vi "LabJack_galvo.vi"() -> ()   [LabVIEW 2025]
uses:
  <vilib>/measure/NI_MABase.lvlib
panel:
  in  "offset":dbl=2.5000000000000013 min=0.0 max=4.5 step=0.1
  in  "stop  2":bool
  in  "stop":bool
  out "DAQ Output Voltage":waveform(dbl)[](graph)
  in  "Waveform Y-Axis":string(combo)="sine"
  in  "Frequency (Hz) 2":i32=20
  in  "Phase (degrees) 2":i32
  in  "Voltage Amplitude 2":dbl=1.0 min=0.0 max=4.5 step=0.1
  in  "Number of Points":dbl=1000.0 format="%#_13g"
  in  "Sampling frequency":dbl=5000.0 format="%#_13g"
  in  "Voltage Amplitude":dbl=1.0 min=0.0 max=4.5 step=0.1
  in  "Phase (degrees)":i32
  in  "Frequency (Hz)":i32=20
  in  "Waveform X-Axis":string(combo)="sine"
  in  "Stream Targets":string[](array[string])=["DAC0", "DAC1"]
  in  "Identifier":string="LJM_idANY"
  in  "ConnectionType":string="LJM_ctANY"
  in  "DeviceType":string="LJM_dtANY"
  out "Error Message":string="No Error"
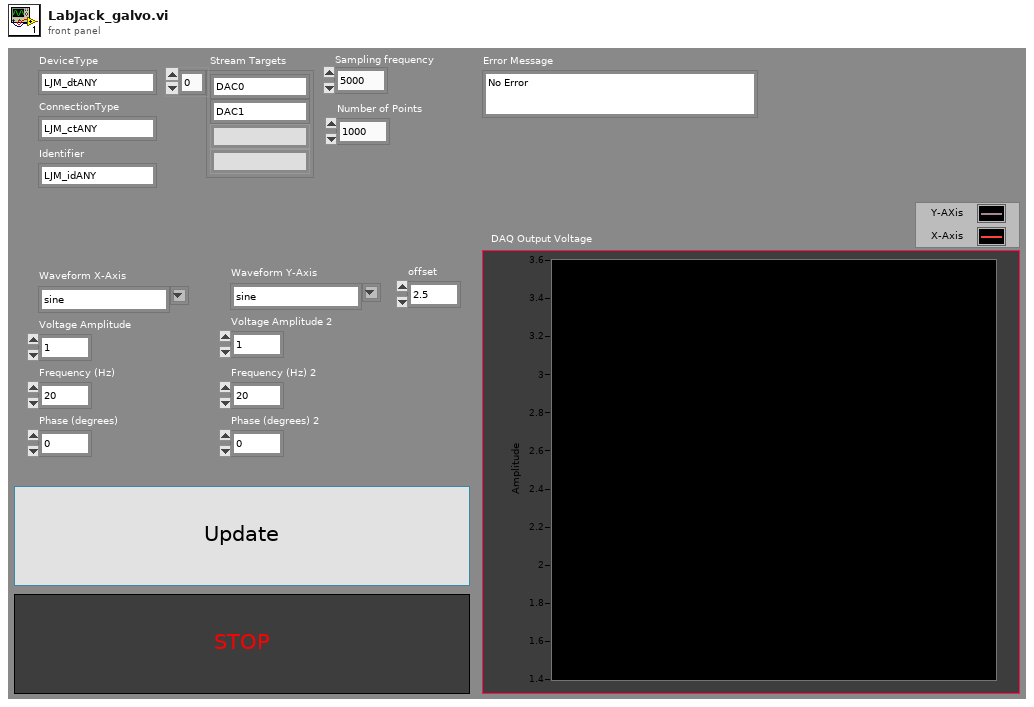
[diagram p1: front panel]
types:
  T1 = cluster{"Sampling frequency":dbl, "Number of Points":dbl}
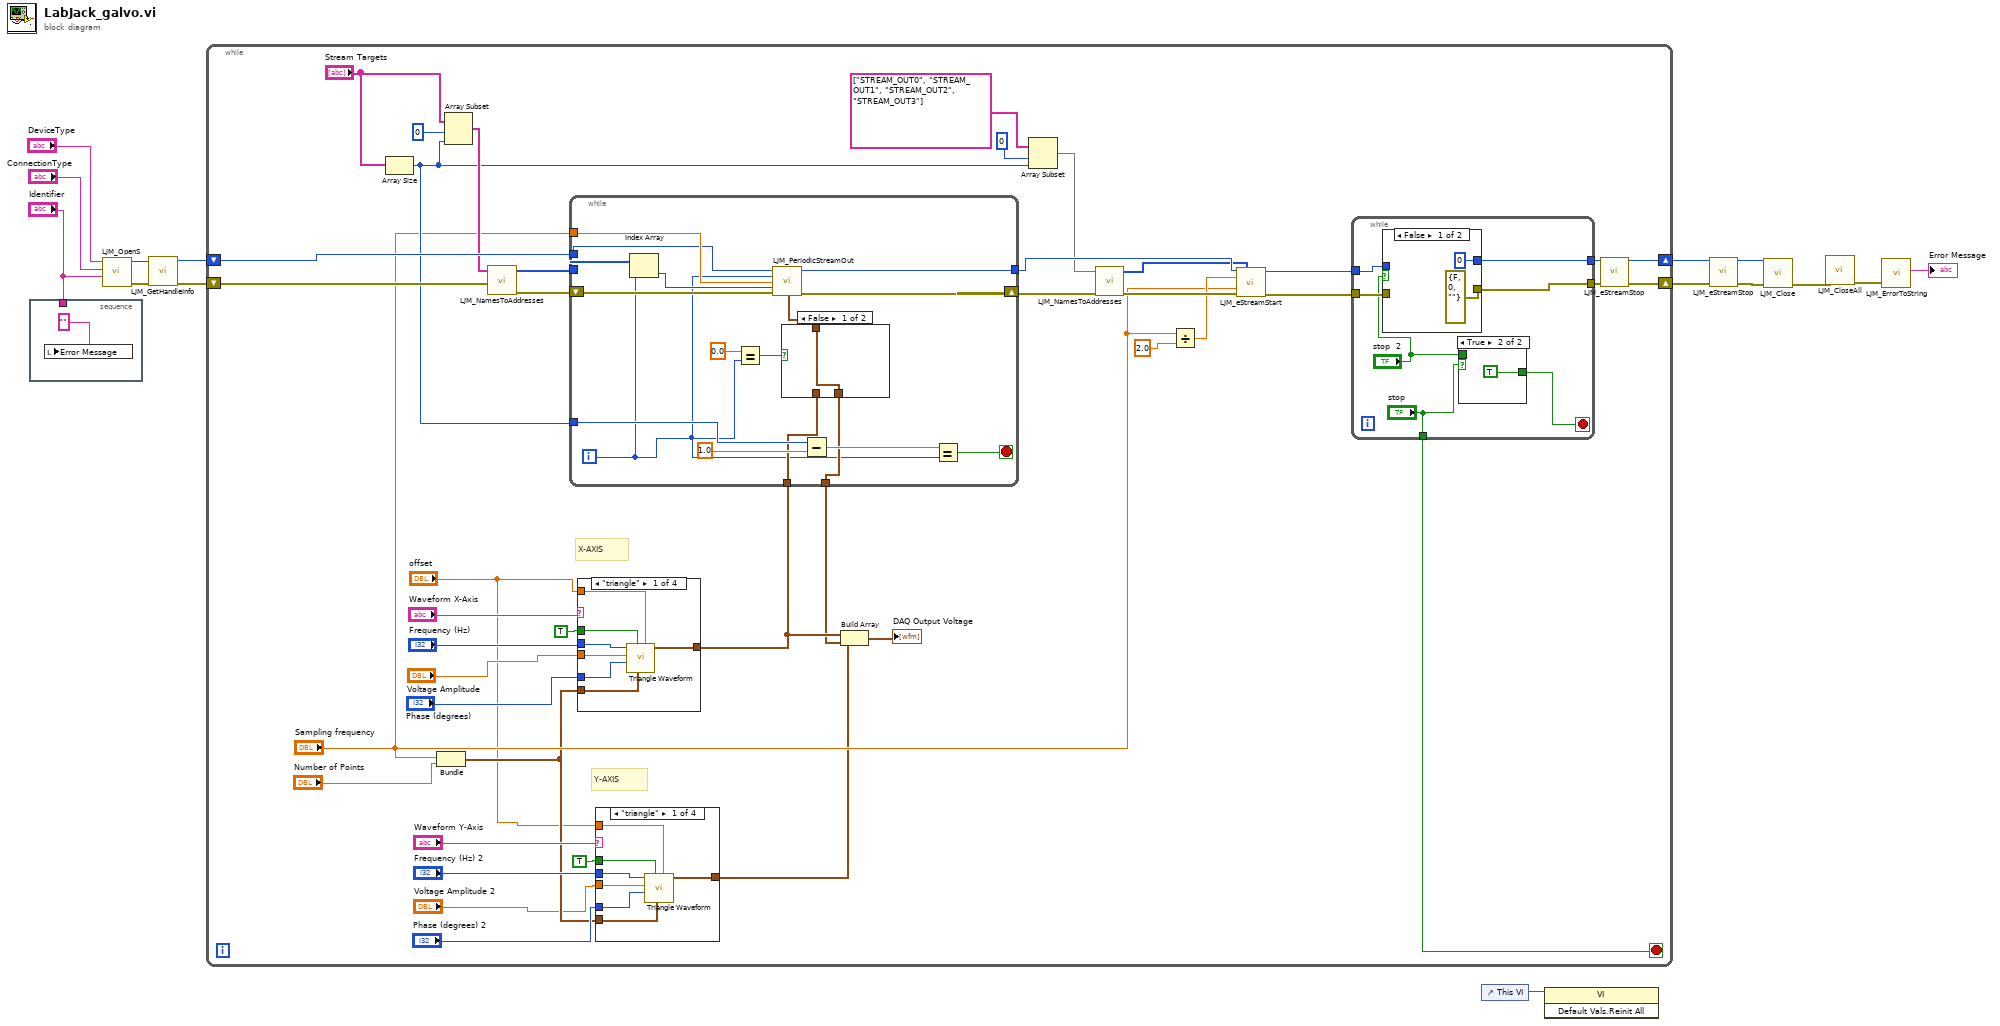
[diagram p0: block diagram]
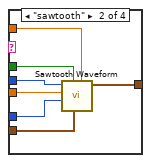
[diagram p4: hidden frame]
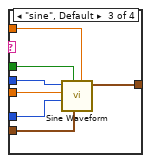
[diagram p5: hidden frame]
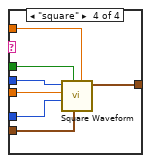
[diagram p6: hidden frame]
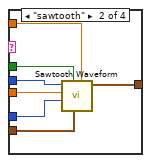
[diagram p7: hidden frame]
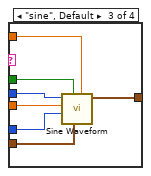
[diagram p8: hidden frame]
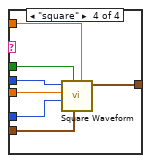
[diagram p9: hidden frame]
diagram:
  n1 = stacked-sequence {
    tunnel: "Identifier" -> [_]
    frame #0 {
      n2 = local write "Error Message"("" ("Error Message")) -> ()
    }
  }
  n3 = call <vilib>:"LJM_OpenS.vi"("Identifier"="Identifier", "ConnectionType"="ConnectionType", "DeviceType"="DeviceType") -> ("error out"=w15:errorcluster, "Handle"=w12:i32)  [unwired: 7 in]
  n4 = call <vilib>:"LJM_GetHandleInfo.vi"("error in"=w15, "Handle In"=w12) -> ("error out"=w9:errorcluster, "Handle Out"=w10:i32)  [unwired: 2 in, 6 out]
  n5 = while {
    shift-right: [w42] -> w4
    shift-left: w10 -> [w56]
    shift-right: [w43] -> w3
    shift-left: w9 -> [w50]
    stop <- w20 stop-if-true
    # "Y-AXIS"
    # "X-AXIS"
    n6 = Array Size(array="Stream Targets") -> (size(s)=w39:i32)
    n7 = Bundle("Sampling frequency"="Sampling frequency", "Number of Points"="Number of Points") -> (w28:T1)  [unwired: 1 in]
    n8 = Array Subset(array="Stream Targets", index=0, length=w39) -> (w53:string[])
    n9 = call <vilib>:"LJM_NamesToAddresses.vi"("error in"=w50, "aNames"=w53) -> ("error out"=w51:errorcluster, "aAddresses"=w52:i32[])  [unwired: 7 in, 1 out]
    n10 = case shown="\"triangle\"" "Waveform X-Axis" {
      tunnel: "Voltage Amplitude" -> [w100 w107 w114 w121]
      tunnel: "Frequency (Hz)" -> [w105 w112 w119 w126]
      tunnel: w28 -> [w102 w109 w117 w125]
      tunnel: [w103 w108 w116 w124] -> w22
      tunnel: "Phase (degrees)" -> [w104 w111 w118 w123]
      tunnel: TRUE ("reset signal") -> [w101 w110 w115 w122]
      tunnel: "offset" -> [w99 w106 w113 w120]
      frame "triangle" {
        n11 = call <vilib>:"Triangle Waveform.vi"("offset"=w99, "sampling info"=w102, "reset signal"=w101, "phase"=w104, "amplitude"=w100, "frequency"=w105) -> ("signal out"=w103:waveform(dbl))  [unwired: 4 in, 1 out]
      }
      frame "sawtooth" {
        n12 = call <vilib>:"Sawtooth Waveform.vi"("offset"=w106, "sampling info"=w109, "reset signal"=w110, "phase"=w111, "amplitude"=w107, "frequency"=w112) -> ("signal out"=w108:waveform(dbl))  [unwired: 4 in, 1 out]
      }
      frame "sine", Default {
        n13 = call <vilib>:"Sine Waveform.vi"("offset"=w113, "sampling info"=w117, "reset signal"=w115, "phase"=w118, "amplitude"=w114, "frequency"=w119) -> ("signal out"=w116:waveform(dbl))  [unwired: 4 in, 1 out]
      }
      frame "square" {
        n14 = call <vilib>:"Square Waveform.vi"("offset"=w120, "sampling info"=w125, "reset signal"=w122, "phase"=w123, "amplitude"=w121, "frequency"=w126) -> ("signal out"=w124:waveform(dbl))  [unwired: 4 in, 1 out]
      }
    }
    n15 = case shown="\"triangle\"" "Waveform Y-Axis" {
      tunnel: "Voltage Amplitude 2" -> [w72 w79 w86 w93]
      tunnel: "Frequency (Hz) 2" -> [w77 w84 w91 w98]
      tunnel: w28 -> [w74 w81 w89 w97]
      tunnel: [w75 w80 w88 w96] -> w21
      tunnel: "Phase (degrees) 2" -> [w76 w83 w90 w95]
      tunnel: TRUE ("reset signal") -> [w73 w82 w87 w94]
      tunnel: "offset" -> [w71 w78 w85 w92]
      frame "triangle" {
        n16 = call <vilib>:"Triangle Waveform.vi"("offset"=w71, "sampling info"=w74, "reset signal"=w73, "phase"=w76, "amplitude"=w72, "frequency"=w77) -> ("signal out"=w75:waveform(dbl))  [unwired: 4 in, 1 out]
      }
      frame "sawtooth" {
        n17 = call <vilib>:"Sawtooth Waveform.vi"("offset"=w78, "sampling info"=w81, "reset signal"=w82, "phase"=w83, "amplitude"=w79, "frequency"=w84) -> ("signal out"=w80:waveform(dbl))  [unwired: 4 in, 1 out]
      }
      frame "sine", Default {
        n18 = call <vilib>:"Sine Waveform.vi"("offset"=w85, "sampling info"=w89, "reset signal"=w87, "phase"=w90, "amplitude"=w86, "frequency"=w91) -> ("signal out"=w88:waveform(dbl))  [unwired: 4 in, 1 out]
      }
      frame "square" {
        n19 = call <vilib>:"Square Waveform.vi"("offset"=w92, "sampling info"=w97, "reset signal"=w94, "phase"=w95, "amplitude"=w93, "frequency"=w98) -> ("signal out"=w96:waveform(dbl))  [unwired: 4 in, 1 out]
      }
    }
    n20 = while {
      tunnel: w39 -> [w133]
      tunnel: w52 -> [w135]
      shift-right: [w140] -> w55
      shift-left: w51 -> [w139]
      tunnel: [w138] -> w48
      tunnel: "Sampling frequency" -> [w137]
      tunnel: w56 -> [w136]
      tunnel: w22 -> [w132]
      tunnel: w21 -> [w131]
      i -> [w128]
      stop <- w143 stop-if-true
      n21 = Index Array(array=w135, index=w128) -> (element=w134:i32)
      n22 = Equal?(x=0.0, y=w128) -> (x = y?=w130:bool)
      n23 = case shown="False" w130 {
        tunnel: w132 -> [_ w145]
        tunnel: w131 -> [w144 _]
        tunnel: [w144 w145] -> w127
        frame False {
        }
        frame True {
        }
      }
      n24 = call <vilib>:"LJM_PeriodicStreamOut.vi"("Handle In"=w136, "Stream-out  Index"=w128, "ScanRate"=w137, "TargetAddr"=w134, "error in"=w139, "aWriteData"=w127) -> ("Handle Out"=w138:i32, "error out"=w140:errorcluster)  [unwired: 8 in]
      n25 = Subtract(x=w133, y=1.0) -> (x-y=w141:dbl)
      n26 = Equal?(x=w141, y=w128) -> (x = y?=w143:bool)
    }
    n27 = Build Array(w22, w21) -> (→"DAQ Output Voltage":waveform(dbl)[])
    n28 = Array Subset(array=string[] ["STREAM_OUT0", "STREAM_OUT1", "STREAM_OUT2", "STREAM_OUT3"], index=0, length=w39) -> (w41:string[])
    n29 = call <vilib>:"LJM_NamesToAddresses.vi"("error in"=w55, "aNames"=w41) -> ("error out"=w47:errorcluster, "aAddresses"=w46:i32[])  [unwired: 7 in, 1 out]
    n30 = Divide(x="Sampling frequency", y=2.0) -> (x/y=w44:dbl)
    n31 = call <vilib>:"LJM_eStreamStart.vi"("Handle In"=w48, "aScanList"=w46, "ScansPerRead"=w44, "ScanRate"="Sampling frequency", "error in"=w47) -> ("Handle Out"=w27:i32, "error out"=w26:errorcluster)  [unwired: 5 in, 4 out]
    n32 = while {
      tunnel: w27 -> [w64]
      tunnel: w26 -> [w62]
      tunnel: [w63] -> w25
      tunnel: [w61] -> w24
      tunnel: ["stop"] -> w20
      stop <- w59 stop-if-true
      n33 = case shown="False" "stop  2" {
        tunnel: w64 -> [_ w70]
        tunnel: [0 ("Handle Out") w70] -> w63
        tunnel: w62 -> [_ w69]
        tunnel: [errorcluster {"status"=FALSE, "code"=0, "source"=""} ("error out") w69] -> w61
        frame False {
        }
        frame True {
        }
      }
      n34 = case shown="True" "stop" {
        tunnel: [w65 TRUE] -> w59
        tunnel: "stop  2" -> [w65 _]
        frame False {
        }
        frame True {
        }
      }
    }
    n35 = call <vilib>:"LJM_eStreamStop.vi"("Handle In"=w25, "error in"=w24) -> ("Handle Out"=w42:i32, "error out"=w43:errorcluster)  [unwired: 12 in]
  }
  n36 = control-ref of="This VI"() -> (w7:refnum<vi>)
  n37 = invoke class="VI" method="Default Vals.Reinit All"(reference=w7) -> ()  [unwired: 2 in, 3 out]
  n38 = call <vilib>:"LJM_eStreamStop.vi"("Handle In"=w4, "error in"=w3) -> ("Handle Out"=w6:i32, "error out"=w5:errorcluster)  [unwired: 12 in]
  n39 = call <vilib>:"LJM_Close.vi"("error in"=w5, "Handle"=w6) -> ("error out"=w2:errorcluster)  [unwired: 9 in]
  n40 = call <vilib>:"LJM_CloseAll.vi"("error in"=w2) -> ("error out"=w1:errorcluster)  [unwired: 10 in]
  n41 = call <vilib>:"LJM_ErrorToString.vi"("error in"=w1) -> ("String"=→"Error Message":string)  [unwired: 10 in]
